vi "TestPFGVPersonnelManagment.vi"() -> (0 "error out":errorcluster, 2 "Pass":bool)   [LabVIEW 2015]
uses:
  TypeDef/PersonnelActions.ctl
  LVClasses/Personnel/PersonnelType.ctl
  LVClasses/Personnel/Personnel.lvclass
panel:
  out "Added":bool
  out "Removed?":bool
  out "DataInit PUIDs":string
  out "Add Personnel 2":string
  out "Read PUIDs 2":string
  out "Remove Personnel":string
  out "Add Personnel":string
  out "Read PUIDS":string
  in  "PUID":string="d1"
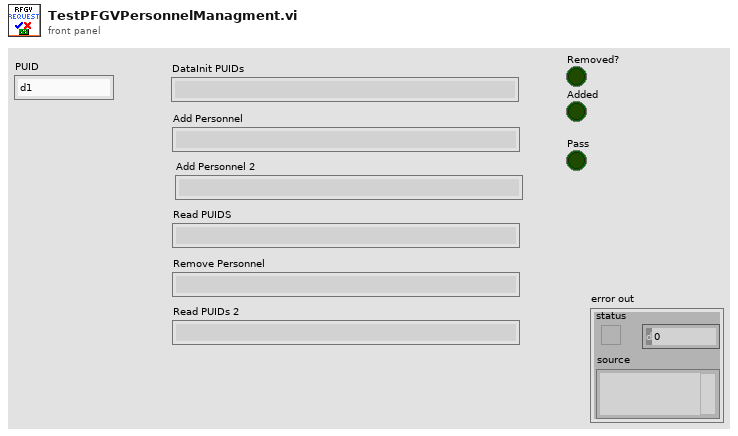
[diagram p1: front panel]
types:
  T1 = typedef "Personnel.lvclass/PersonnelType.ctl" = enum16{"Nurse", "Doctor", "Cleanning", "Admin"}
  T2 = typedef "PersonnelActions.ctl" = enum16{"Init", "Read Personnel", "Add Personnel", "Remove Personnel", "Read Name", "Write Name", "Read Role", "Write Role", "Read Requests", "Add Requests", "Remove Requests", "Read PUIDs"}
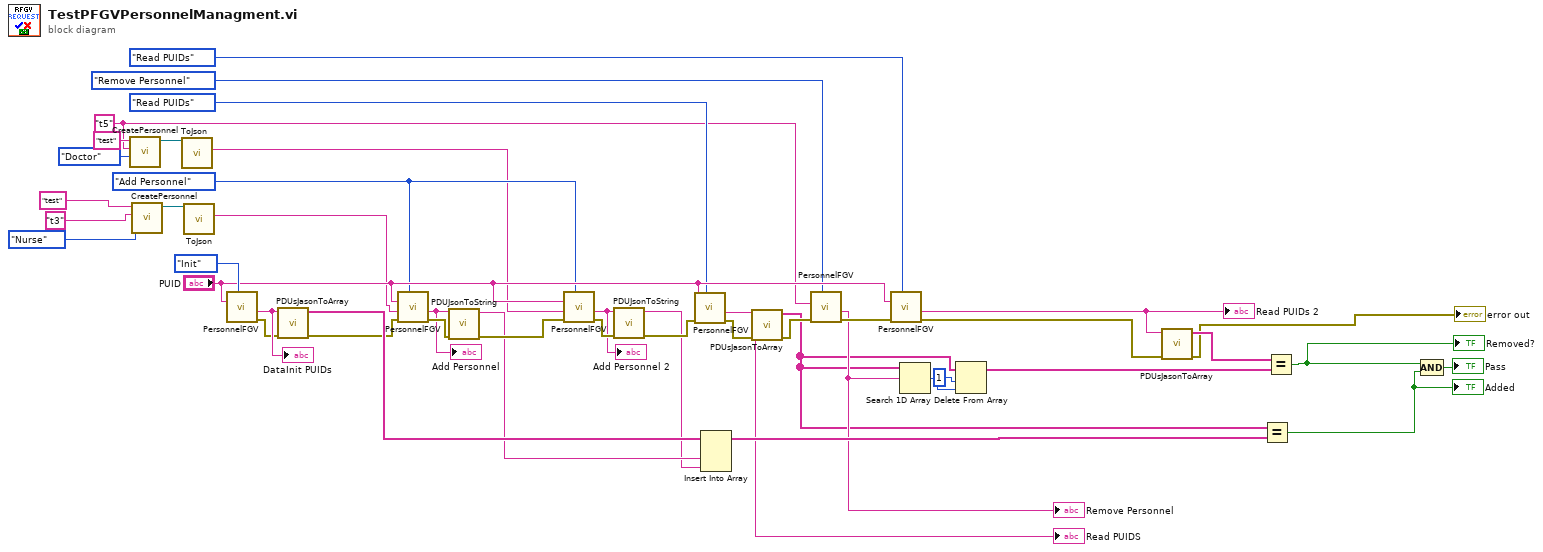
[diagram p0: block diagram]
diagram:
  w2 = "t5" ("UniqueID")
  w37 = PersonnelActions."Add Personnel" ("Actions")
  n1 = call "CreatePersonnel.vi"("Role"=PersonnelType."Doctor", "UniqueID"=w2, "Name"="test") -> ("output cluster"=w36:refnum<class "Personnel.lvclass">)  [unwired: 7 in, 1 out]
  n2 = call "CreatePersonnel.vi"("Role"=PersonnelType."Nurse", "UniqueID"="t3", "Name"="test") -> ("output cluster"=w35:refnum<class "Personnel.lvclass">)  [unwired: 7 in, 1 out]
  n3 = call "ToJson.vi"("Personnel in"=w36) -> ("PersonnelJson"=w3:string)  [unwired: 8 in, 2 out]
  n4 = call "ToJson.vi"("Personnel in"=w35) -> ("PersonnelJson"=w34:string)  [unwired: 8 in, 2 out]
  n5 = call "PersonnelFGV.vi"("Actions"=PersonnelActions."Init", "PUID"="PUID") -> ("error out"=w25:errorcluster, "Data Out"=w28:string)  [unwired: 8 in]
  "DataInit PUIDs" <- w28
  n6 = call "PDUsJasonToArray.vi"("error in (no error)"=w25, "Data Out"=w28) -> ("error out"=w24:errorcluster, "PUIDs"=w26:string[])  [unwired: 8 in]
  n7 = call "PersonnelFGV.vi"("Actions"=w37, "error in (no error)"=w24, "Data In"=w34, "PUID"="PUID") -> ("error out"=w20:errorcluster, "Data Out"=w13:string)  [unwired: 6 in]
  "Add Personnel" <- w13
  n8 = call "PDUJsonToString.vi"("error in (no error)"=w20, "Data Out"=w13) -> ("error out"=w19:errorcluster, "PUID"=w11:string)  [unwired: 8 in]
  n9 = call "PersonnelFGV.vi"("Actions"=w37, "error in (no error)"=w19, "Data In"=w3, "PUID"="PUID") -> ("error out"=w18:errorcluster, "Data Out"=w12:string)  [unwired: 6 in]
  "Add Personnel 2" <- w12
  n10 = call "PDUJsonToString.vi"("error in (no error)"=w18, "Data Out"=w12) -> ("error out"=w17:errorcluster, "PUID"=w10:string)  [unwired: 8 in]
  n11 = call "PersonnelFGV.vi"("Actions"=PersonnelActions."Read PUIDs", "error in (no error)"=w17, "PUID"="PUID") -> ("error out"=w16:errorcluster, "Data Out"=w9:string)  [unwired: 7 in]
  "Read PUIDS" <- w9
  n12 = Insert Into Array(array=w26, new element #1=w11, new element #2=w10) -> (w27:string[])  [unwired: 1 in]
  n13 = call "PDUsJasonToArray.vi"("error in (no error)"=w16, "Data Out"=w9) -> ("error out"=w15:errorcluster, "PUIDs"=w5:string[])  [unwired: 8 in]
  n14 = call "PersonnelFGV.vi"("Actions"=PersonnelActions."Remove Personnel", "error in (no error)"=w15, "PUID"=w2) -> ("error out"=w14:errorcluster, "Data Out"=w8:string)  [unwired: 7 in]
  "Remove Personnel" <- w8
  n15 = call "PersonnelFGV.vi"("Actions"=PersonnelActions."Read PUIDs", "error in (no error)"=w14, "PUID"="PUID") -> ("error out"=w22:errorcluster, "Data Out"=w23:string)  [unwired: 7 in]
  "Read PUIDs 2" <- w23
  n16 = Search 1D Array(1D array=w5, element=w8) -> (index of element=w7:i32)  [unwired: 1 in]
  n17 = Delete From Array(array=w5, length=1, index=w7) -> (array with subset deleted=w4:string[])  [unwired: 1 out]
  n18 = call "PDUsJasonToArray.vi"("error in (no error)"=w22, "Data Out"=w23) -> ("error out"=→"error out":errorcluster, "PUIDs"=w21:string[])  [unwired: 8 in]
  n19 = Equal?(x=w5, y=w27) -> (x = y?=w43:bool)
  "Added" <- w43
  n20 = Equal?(x=w21, y=w4) -> (x = y?=w45:bool)
  "Removed?" <- w45
  n21 = Compound Arithmetic op=AND(w45, w43) -> (→"Pass":bool)
